vi "Stop.vi"(8 "error in (no error)":errorcluster caption="entrée d'erreur (pas d'erreur)", 11 "DAQmxTaskContainer en entrée":refnum<class "DAQmxTaskContainer.lvclass">) -> (0 "error out":errorcluster caption="sortie d'erreur", 3 "DAQmxTaskContainer en sortie":refnum<class "DAQmxTaskContainer.lvclass">)   [LabVIEW 2015, in "DAQmxTaskContainer.lvclass"]
uses:
  DAQmxTaskContainer.lvclass
  dependecies/ControlsVIs/Clusters-def/SERVER-Commands.ctl
  dependecies/ControlsVIs/Clusters-def/Message types.ctl
  DAQmxTaskContainer_General/DAQmxTaksContainer_General.lvclass/DAQmxTaksContainer_General.ctl
  DAQmxTask.lvclass
  Control/Control-Server/Control-Server.lvclass
  Message/Message.lvclass
  GeneralFunctionality/GeneralFunctionality.lvclass
  DAQmxTaskContainer_General/DAQmxTaksContainer_General.lvclass
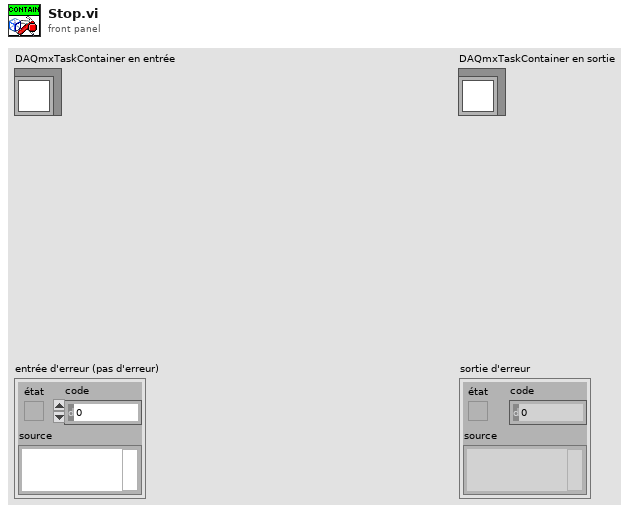
[diagram p1: front panel]
types:
  T1 = typedef "Message types.ctl" = string
  T2 = typedef "Control-Server.lvclass/SERVER-Commands.ctl" = string
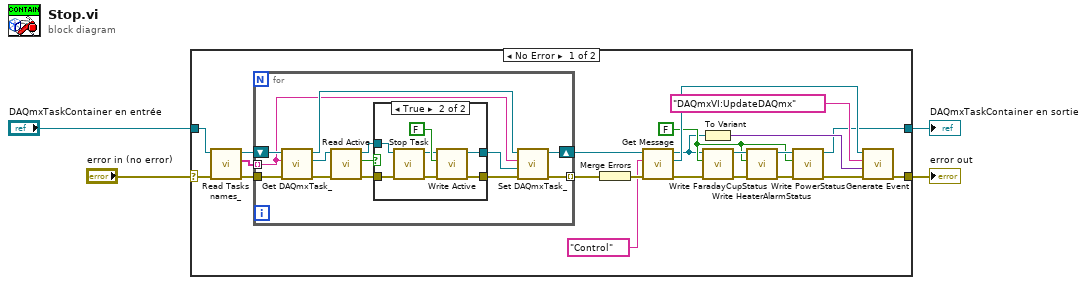
[diagram p0: block diagram]
diagram:
  n1 = case shown="No Error" "error in (no error)" {
    selector: "error in (no error)" -> [w9 w50]
    tunnel: [w24 w50] -> w3
    tunnel: [w13 w49] -> w1
    tunnel: "DAQmxTaskContainer en entrée" -> [w6 w49]
    frame No Error {
      w14 = FALSE ("PowerStatus")
      n2 = call "Read Tasks names_.vi"("error in (no error)"=w9, "DAQmxTaksContainer_General in"=w6) -> ("error out"=w8:errorcluster, "Tasks names"=w7:string[], "DAQmxTaksContainer_General out"=w5:refnum<class "DAQmxTaskContainer.lvclass">)  [unwired: 7 in]
      n3 = for {
        tunnel: w7 -> [w31] mode=indexing
        tunnel: w8 -> [w35]
        tunnel: [w30] -> w26 mode=indexing
        shift-right: [w28] -> w23
        shift-left: w5 -> [w36]
        n4 = call "Get DAQmxTask_.vi"("error in (no error)"=w35, "Task name"=w31, "DAQmxTaksContainer_General in"=w36) -> ("error out"=w33:errorcluster, "DAQmx Task"=w34:refnum<class "DAQmxTask.lvclass">, "DAQmxTaksContainer_General out"=w32:refnum<class "DAQmxTaskContainer.lvclass">)  [unwired: 6 in]
        n5 = call-dynamic "Read Active.vi"("error in (no error)"=w33, "DAQmxTask in"=w34) -> ("error out"=w37:errorcluster, "Active?"=w39:bool, "DAQmxTask out"=w38:refnum<class "DAQmxTask.lvclass">)  [unwired: 7 in]
        n6 = case shown="True" w39 {
          tunnel: w38 -> [w41 w48]
          tunnel: w37 -> [w40 w47]
          tunnel: [w40 w42] -> w29
          tunnel: [w41 w43] -> w27
          frame False {
          }
          frame True {
            n7 = call "Stop Task.vi"("error in (no error)"=w47, "DAQmxTask in"=w48) -> ("error out"=w44:errorcluster, "DAQmxTask out"=w45:refnum<class "DAQmxTask.lvclass">)  [unwired: 8 in]
            n8 = call-dynamic "Write Active.vi"("error in (no error)"=w44, "Active?"=FALSE, "DAQmxTask in"=w45) -> ("error out"=w42:errorcluster, "DAQmxTask out"=w43:refnum<class "DAQmxTask.lvclass">)  [unwired: 7 in]
          }
        }
        n9 = call "Set DAQmxTask_.vi"("error in (no error)"=w29, "DAQmxTask"=w27, "Task name"=w31, "DAQmxTaksContainer_General in"=w32) -> ("error out"=w30:errorcluster, "DAQmxTaksContainer_General out"=w28:refnum<class "DAQmxTaskContainer.lvclass">)  [unwired: 6 in]
      }
      n10 = Merge Errors(w26) -> (w25:errorcluster)
      n11 = call "Get Message.vi"("error in (no error)"=w25, "Message type"=T1 "Control", "GeneralFunctionality en entrée"=w23) -> ("error out"=w11:errorcluster, "Message.lvclass"=w20:refnum<class "Message.lvclass">, "GeneralFunctionality en sortie"=w12:refnum<class "DAQmxTaskContainer.lvclass">)  [unwired: 6 in]
      n12 = To Variant(anything=w12) -> (Variant=w21:variant)
      n13 = call "Write FaradayCupStatus.vi"("error in (no error)"=w11, "FaradayCupStatus"=w14, "DAQmxTaksContainer_General in"=w12) -> ("error out"=w15:errorcluster, "DAQmxTaksContainer_General out"=w16:refnum<class "DAQmxTaskContainer.lvclass">)  [unwired: 7 in]
      n14 = call "Write HeaterAlarmStatus.vi"("error in (no error)"=w15, "HeaterAlarmStatus"=w14, "DAQmxTaksContainer_General in"=w16) -> ("error out"=w17:errorcluster, "DAQmxTaksContainer_General out"=w18:refnum<class "DAQmxTaskContainer.lvclass">)  [unwired: 7 in]
      n15 = call "Write PowerStatus.vi"("error in (no error)"=w17, "PowerStatus"=w14, "DAQmxTaksContainer_General in"=w18) -> ("error out"=w10:errorcluster, "DAQmxTaksContainer_General out"=w13:refnum<class "DAQmxTaskContainer.lvclass">)  [unwired: 7 in]
      n16 = call "Generate Event.vi"("error in (no error)"=w10, "Data"=w21, "Command"=T2 "DAQmxVI:UpdateDAQmx", "Message en entrée"=w20) -> ("error out"=w24:errorcluster)  [unwired: 6 in, 1 out]
    }
    frame Error {
    }
  }
  "error out" <- w3
  "DAQmxTaskContainer en sortie" <- w1
